vi "Ignore nearby.vi"(2 "Particle Measurements (Real-World) (Particle Analysis 1)":dbl[][](array[numeric])) -> (0 "s? t:f":dbl[][](array[numeric]), 1 "appended array":dbl[][](array[numeric]))   [LabVIEW 2022 SP3]
doc: "This Vi removes from object array if they are closer together than 5mm"
panel:
  out "Array":dbl[][](array[numeric])
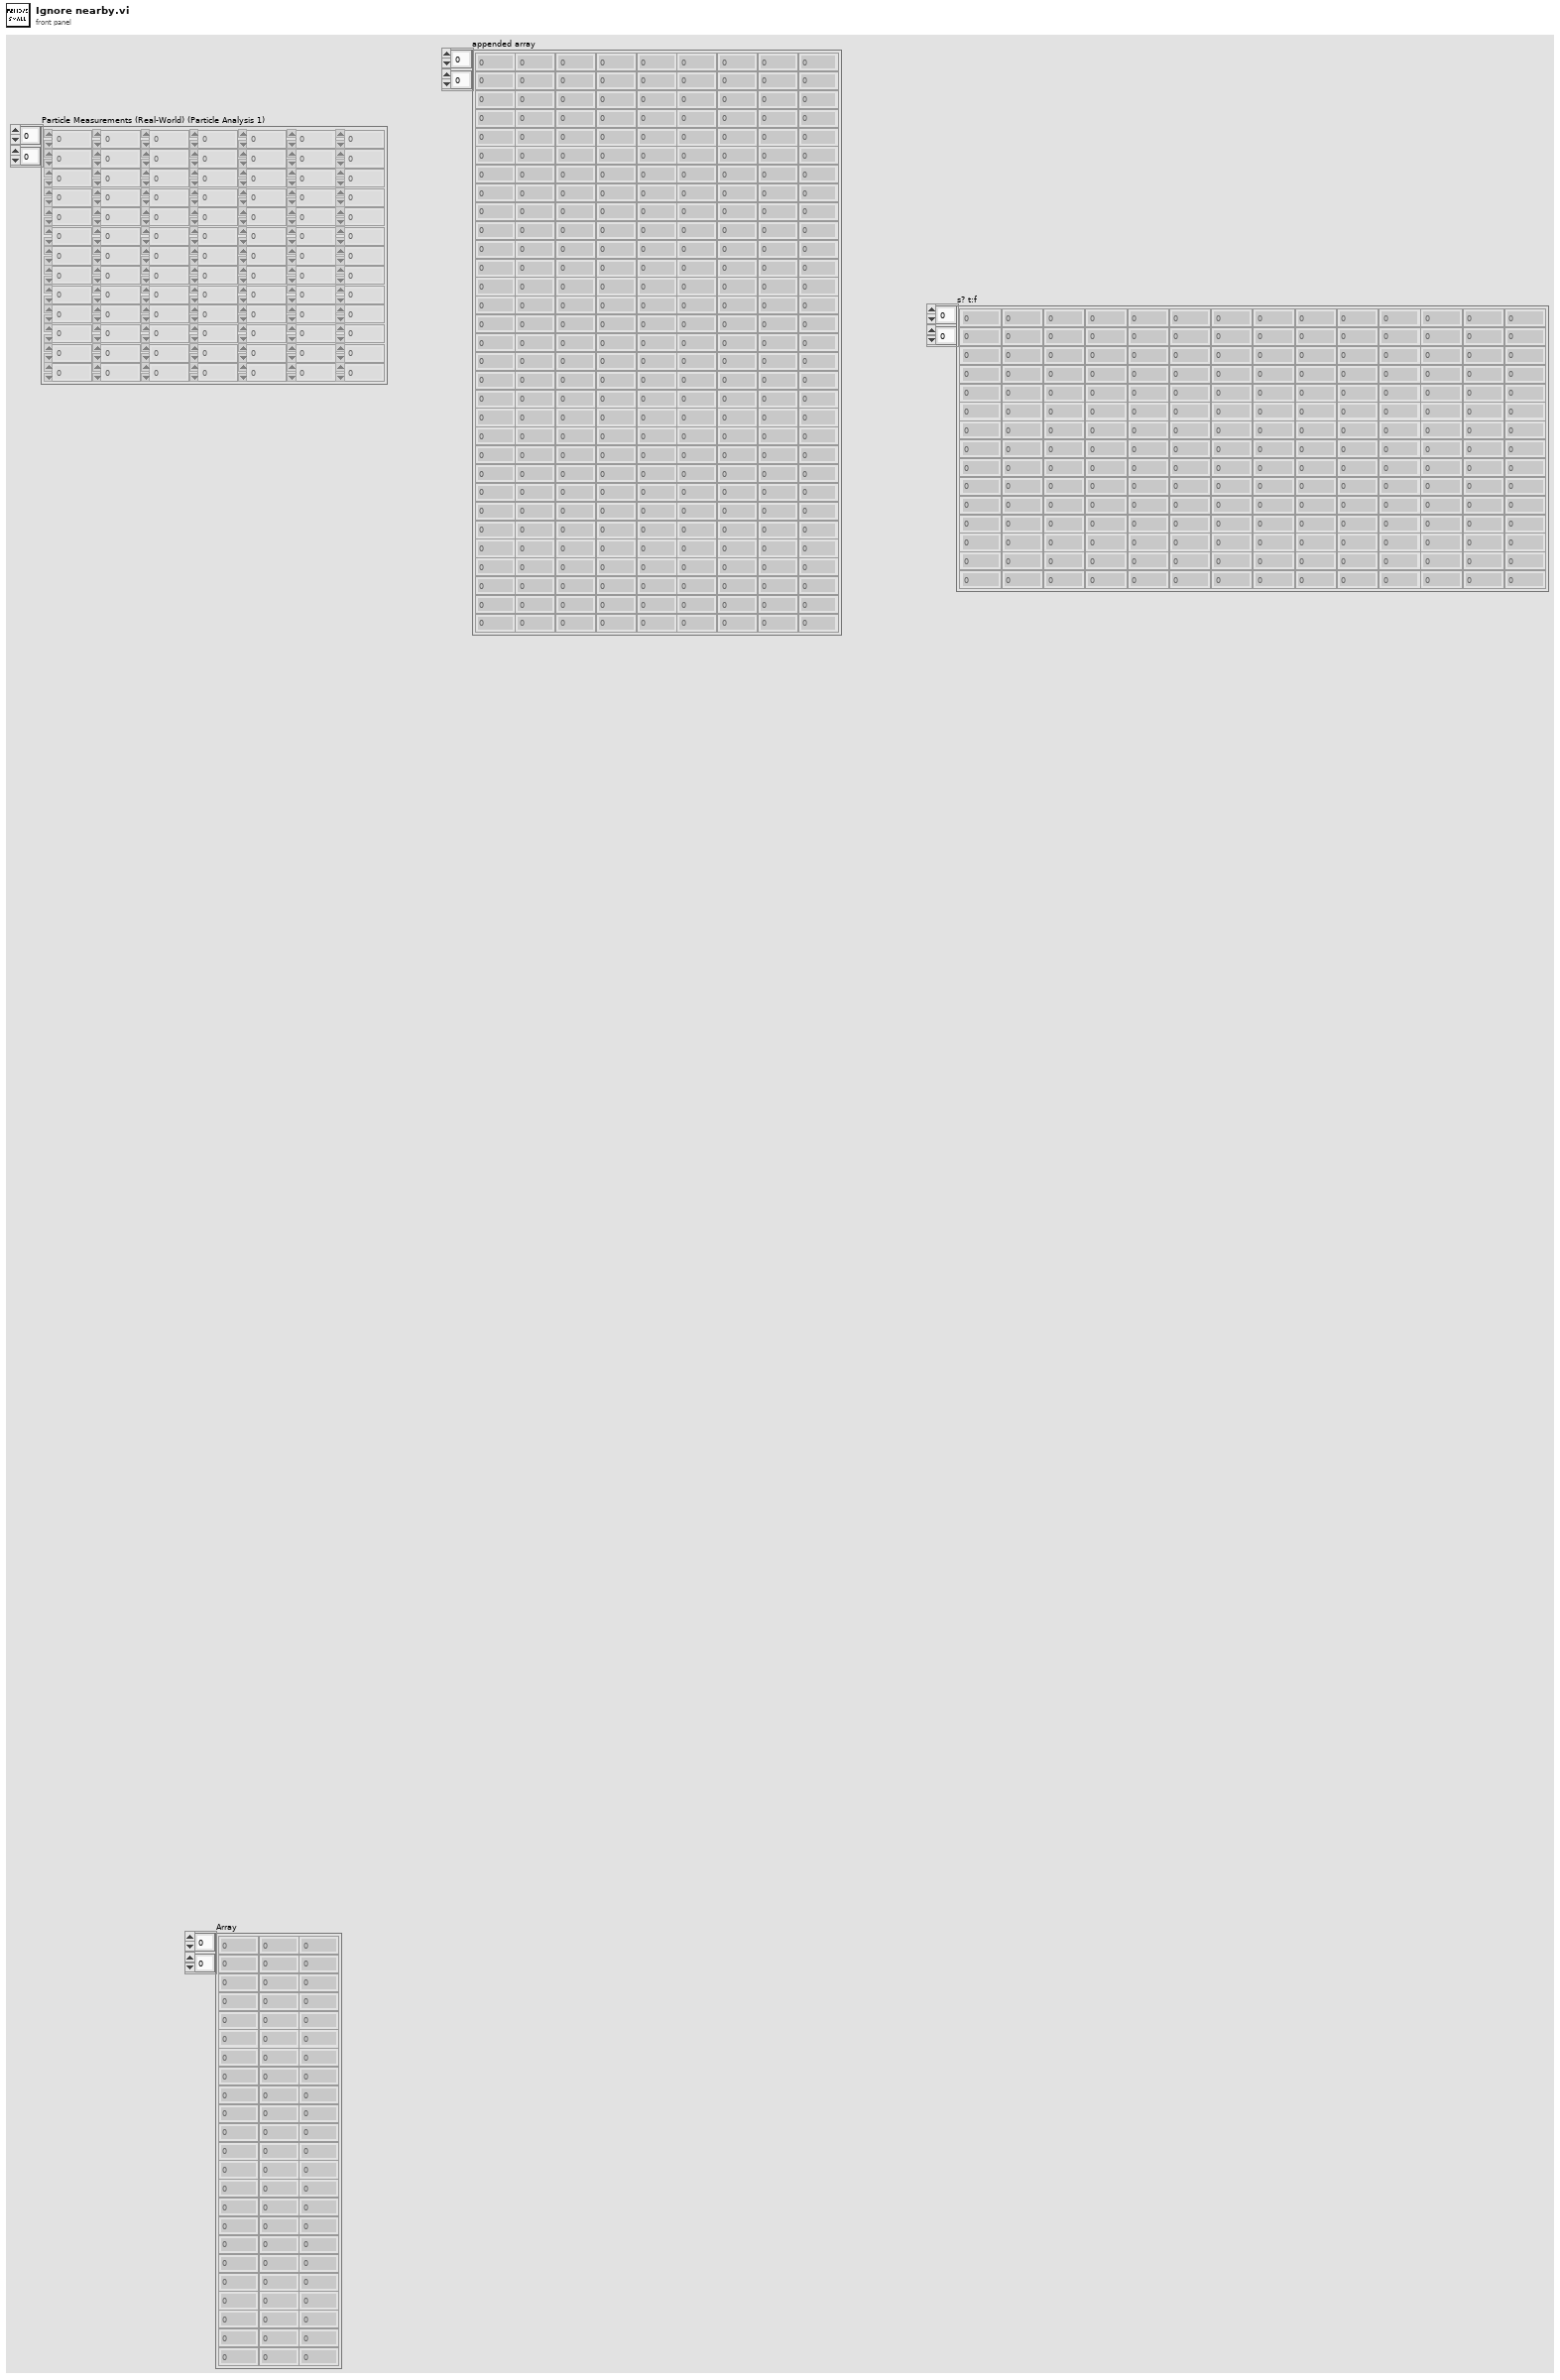
[diagram p1: front panel]
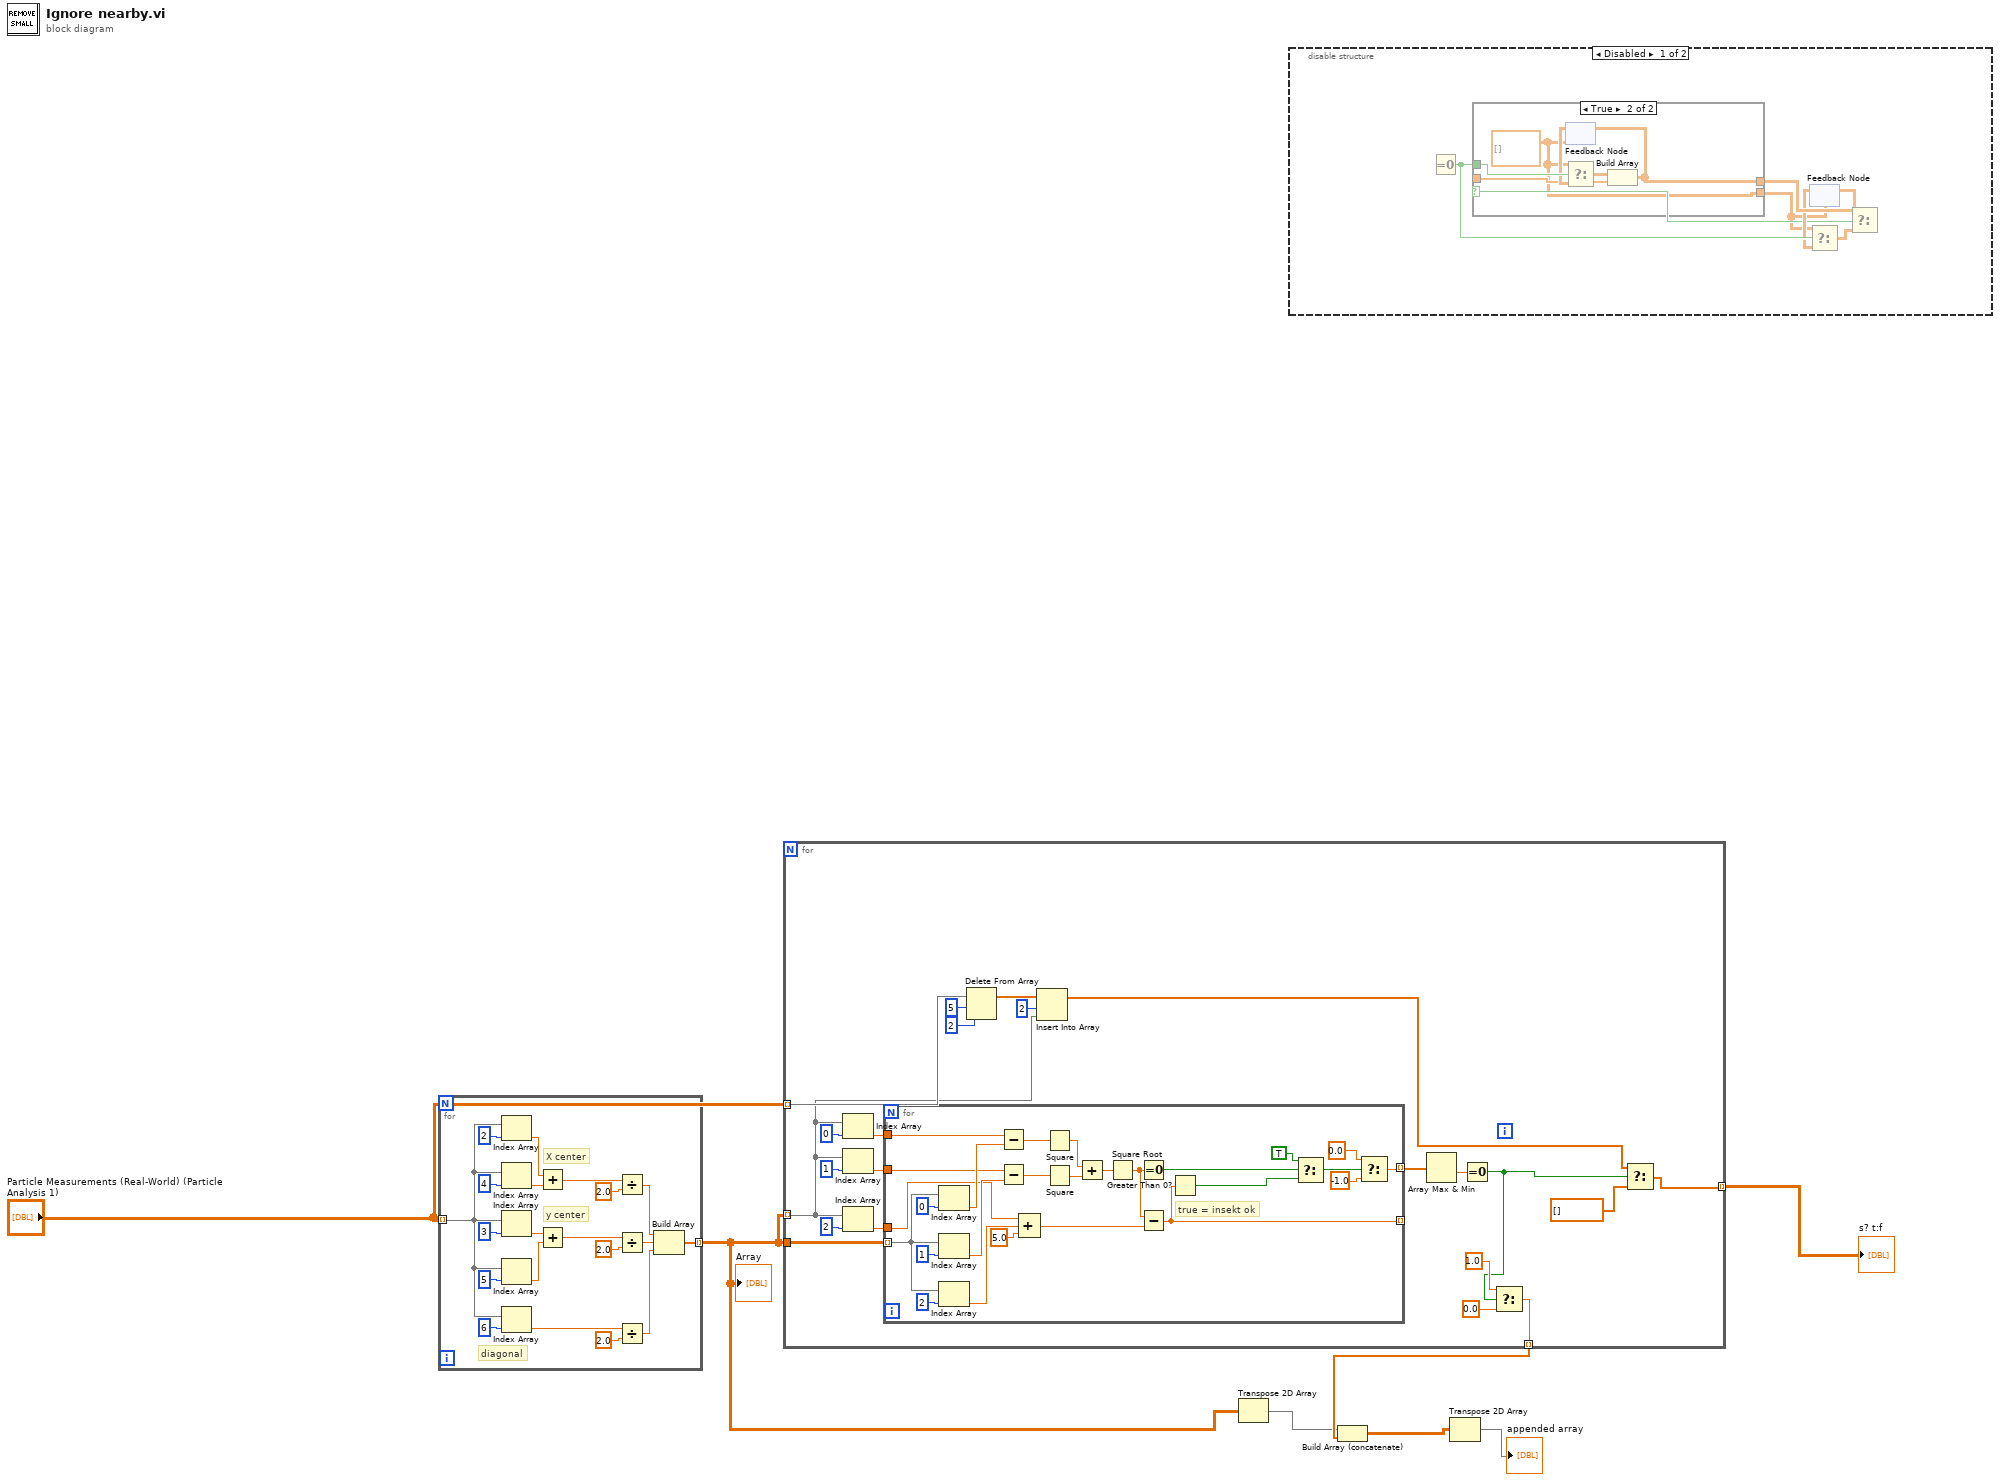
[diagram p0: block diagram]
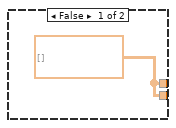
[diagram p2: hidden frame]
diagram:
  n1 = for {
    tunnel: "Particle Measurements (Real-World) (Particle Analysis 1)" -> [w14] mode=indexing
    tunnel: [w12] -> w5 mode=indexing
    # "diagonal"
    # "y center"
    # "X center"
    n2 = Index Array(array=w14, index=2 ("index (row)")) -> (element=w22:dbl)
    n3 = Index Array(array=w14, index=4 ("index (row)")) -> (element=w25:dbl)
    n4 = Index Array(array=w14, index=3 ("index (row)")) -> (element=w21:dbl)
    n5 = Index Array(array=w14, index=5 ("index (row)")) -> (element=w18:dbl)
    n6 = Index Array(array=w14, index=6 ("index (row)")) -> (element=w9:dbl)
    n7 = Add(x=w22, y=w25) -> (x+y=w24:dbl)
    n8 = Add(x=w21, y=w18) -> (x+y=w19:dbl)
    n9 = Divide(x=w24, y=2.0) -> (x/y=w13:dbl)
    n10 = Divide(x=w19, y=2.0) -> (x/y=w11:dbl)
    n11 = Divide(x=w9, y=2.0) -> (x/y=w8:dbl)
    n12 = Build Array(w13, w11, w8) -> (w12:dbl[])
  }
  "Array" <- w5
  n13 = for {
    tunnel: w5 -> [w35] mode=indexing
    tunnel: w5 -> [w46]
    tunnel: "Particle Measurements (Real-World) (Particle Analysis 1)" -> [w37] mode=indexing
    tunnel: [w29] -> w7 mode=indexing
    tunnel: [w38] -> w6 mode=indexing
    n14 = Index Array(array=w35, index=0 ("index (row)")) -> (element=w45:dbl)
    n15 = Index Array(array=w35, index=1 ("index (row)")) -> (element=w44:dbl)
    n16 = Index Array(array=w35, index=2) -> (element=w43:dbl)
    n17 = for {
      tunnel: w46 -> [w72] mode=indexing
      tunnel: w45 -> [w71]
      tunnel: w44 -> [w68]
      tunnel: w43 -> [w62]
      tunnel: [w57] -> _ mode=indexing
      tunnel: [w50] -> w41 mode=indexing
      # "true = insekt ok"
      n18 = Index Array(array=w72, index=0 ("index (row)")) -> (element=w70:dbl)
      n19 = Index Array(array=w72, index=1 ("index (row)")) -> (element=w67:dbl)
      n20 = Index Array(array=w72, index=2) -> (element=w61:dbl)
      n21 = Subtract(x=w71, y=w70) -> (x-y=w69:dbl)
      n22 = Subtract(x=w68, y=w67) -> (x-y=w66:dbl)
      n23 = Compound Arithmetic op=ADD(w62, w61, 5.0 ("value")) -> (w59:dbl)
      n24 = Square(x=w69) -> (x^2=w65:dbl)
      n25 = Square(x=w66) -> (x^2=w64:dbl)
      n26 = Add(x=w65, y=w64) -> (x+y=w63:dbl)
      n27 = Square Root(x=w63) -> (sqrt(x)=w58:dbl)
      n28 = Equal To 0?(x=w58) -> (x = 0?=w56:bool)
      n29 = Subtract(x=w58, y=w59) -> (x-y=w57:dbl)
      n30 = Greater Than 0?(x=w57) -> (x > 0?=w55:bool)
      n31 = Select(t=TRUE, s=w56, f=w55) -> (s? t:f=w53:bool)
      n32 = Select(t=0.0, s=w53, f=-1.0) -> (s? t:f=w50:dbl)
    }
    n33 = Delete From Array(array=w37, length=5, index=2) -> (array with subset deleted=w36:dbl[])  [unwired: 1 out]
    n34 = Insert Into Array(array=w36, index=2, new element=w35) -> (w30:dbl[])
    n35 = Array Max & Min(array=w41) -> (min value=w42:dbl)  [unwired: 3 out]
    n36 = Equal To 0?(x=w42) -> (x = 0?=w31:bool)
    n37 = Select(t=1.0, s=w31, f=0.0) -> (s? t:f=w38:dbl)
    n38 = Select(t=w30, s=w31, f=dbl[] []) -> (s? t:f=w29:dbl[])
  }
  "s? t:f" <- w7
  n39 = Transpose 2D Array(2D array=w5) -> (transposed array=w4:dbl[][])
  n40 = disable-structure shown="Disabled" {
    frame Disabled {
      n41 = Equal To 0?() -> (x = 0?=w81:bool)  [unwired: 1 in]
      n42 = case shown="True" w77 {
        tunnel: w81 -> [_ w89]
        tunnel: _ -> [_ w86]
        tunnel: [w83 w85] -> w82
        tunnel: [w83 w84] -> w76
        frame False {
          w83 = dbl[][] []
        }
        frame True {
          w84 = dbl[][] []
          n43 = feedback #1(w84) -> (w87:dbl[][])
          n44 = Select(t=w84, s=w89, f=w87) -> (s? t:f=w88:dbl[][])
          n45 = Build Array(w88, w86) -> (w85:dbl[][][])
          n46 = feedback-in #1(w85) -> ()
        }
      }
      n47 = feedback #2(w76) -> (w80:dbl[][])
      n48 = Select(t=w76, s=w81, f=w80) -> (s? t:f=w79:dbl[][])
      n49 = Select(t=w82, f=w79) -> (s=w77:bool, s? t:f=w78:dbl[][][])
      n50 = feedback-in #2(w78) -> ()
    }
    frame Enabled {
    }
  }
  n51 = Build Array (concatenate)(w4, w6) -> (w2:dbl[][])
  n52 = Transpose 2D Array(2D array=w2) -> (transposed array=→"appended array":dbl[][])
